vi "ChangeTblBgColor.vi"(6 "reference":refnum<vi>, 7 "Row":i32, 8 "input string":string) -> (3 "Color":u32)   [LabVIEW 2019]
uses:
  <vilib>/Utility/miscctls.llb/LVRowAndColumnTypeDef.ctl
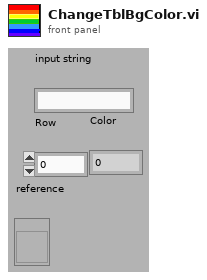
[diagram p1: front panel]
types:
  T1 = typedef "LVRowAndColumnTypeDef.ctl" = cluster{"Row":i32, "Column":i32}
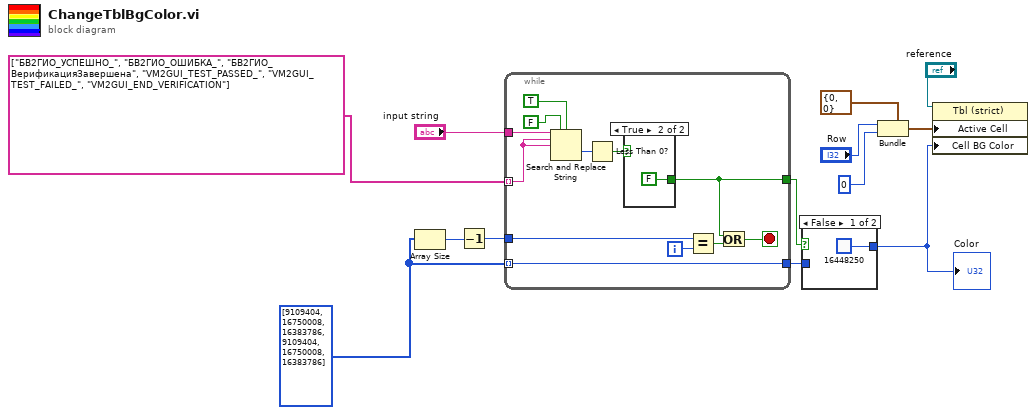
[diagram p0: block diagram]
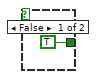
[diagram p3: hidden frame]
diagram:
  w12 = u32[] [9109404, 16750008, 16383786, 9109404, 16750008, 16383786]
  n1 = Array Size(array=w12) -> (size(s)=w8:i32)
  n2 = Decrement(x=w8) -> (x-1=w7:i32)
  n3 = while {
    tunnel: string[] ["БВ2ГИО_УСПЕШНО_", "БВ2ГИО_ОШИБКА_", "БВ2ГИО_ВерификацияЗавершена", "VM2GUI_TEST_PASSED_", "VM2GUI_TEST_FAILED_", "VM2GUI_END_VERIFICATION"] -> [w22] mode=indexing
    tunnel: "input string" -> [w21]
    tunnel: w12 -> [w14] mode=indexing
    tunnel: w7 -> [w19]
    tunnel: [w15] -> w6
    tunnel: [w14] -> w5
    i -> [w16]
    stop <- w17 stop-if-true
    n4 = Search and Replace String(replace all?=FALSE ("replace all? (F)"), case sensitive?=TRUE ("ignore case? (F)"), input string=w21, search string=w22, replace string=w22) -> (offset past replacement=w23:i32)  [unwired: 3 in, 3 out]
    n5 = Less Than 0?(x=w23) -> (x < 0?=w20:bool)
    n6 = case shown="True" w20 {
      tunnel: [TRUE FALSE] -> w15
      frame False {
      }
      frame True {
      }
    }
    n7 = Equal?(x=w19, y=w16) -> (x = y?=w18:bool)
    n8 = Or(x=w15, y=w18) -> (x .or. y?=w17:bool)
  }
  n9 = case shown="False" w6 {
    tunnel: w5 -> [_ w29]
    tunnel: [u32 16448250 ("Success") w29] -> w2
    frame False {
    }
    frame True {
    }
  }
  "Color" <- w2
  n10 = Bundle(cluster=T1 {"Row"=0, "Column"=0} ("Active Cell:Active Cell"), "Row"="Row", "Column"=0) -> (w3:T1)
  n11 = property class="Tbl (strict)"(reference="reference", "Active Cell"=w3, "Cell BG Color"=w2) -> ()  [unwired: 1 in, 2 out]
